vi "snap方式图像采集 1.vi"(8 "error in (no error)":errorcluster caption="错误输入（无错误）", 9 "Session In":T1, 10 "Image Name":string="I1") -> (0 "error out":errorcluster caption="错误输出", 2 "Session Out":T1, 3 "Image out":T2(plugin-control))   [LabVIEW 2017]
uses:
  <vilib>/userdefined/High Color/IMAQdx.ctl
  <vilib>/vision/driver/IMAQdx.llb/IMAQdx Camera Control Mode.ctl
  <vilib>/vision/driver/NI_Vision_Acquisition_Software.lvlib
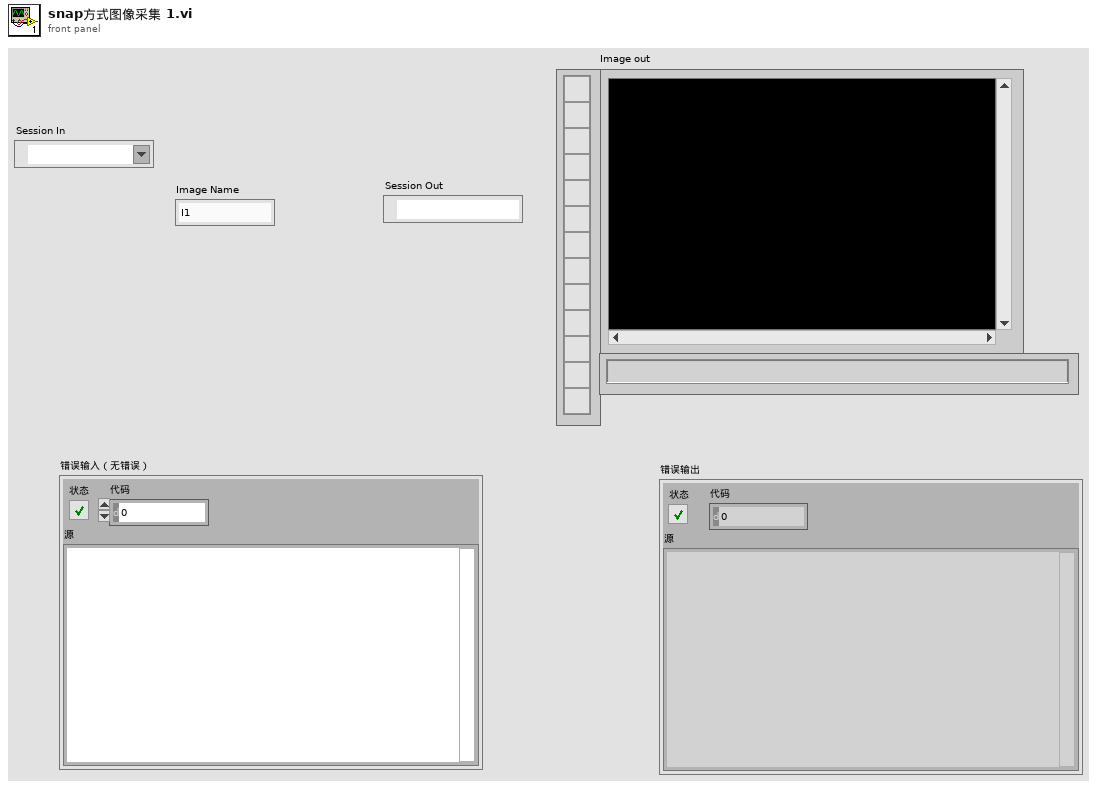
[diagram p1: front panel]
types:
  T1 = typedef "IMAQdx.ctl" = refnum<k21>
  T2 = typedef "IMAQ Image.ctl" = refnum<image>
  T3 = typedef "NI_Vision_Acquisition_Software.lvlib/IMAQdx Camera Control Mode.ctl" = enum32{"Controller", "Listener"}
  T4 = typedef "Image Type" = u32
  T5 = cluster{"IsNorImage":bool, "Exposure Values":u32, "ImagePath":path}
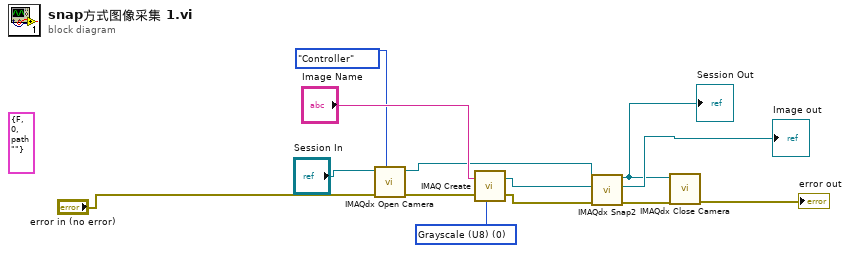
[diagram p0: block diagram]
diagram:
  w11 = T4 0 items=["Grayscale (U8)", "Grayscale (I16)", "Grayscale (SGL)", "Complex (CSG)", "RGB (U32)", "HSL (U32)", "RGB (U64)", "Grayscale (U16)"] ("Image Type")
  (unwired) T5 {"IsNorImage"=FALSE, "Exposure Values"=0, "ImagePath"=path ""} ("ParamsUI")
  n1 = call <vilib>:"IMAQdx Open Camera.vi"("Camera Control Mode"=IMAQdx_Camera_Control_Mode."Controller", "error in"="error in (no error)", "Session In"="Session In") -> ("error out"=w3:errorcluster, "Session Out"=w9:T1)  [unwired: 7 in]
  n2 = call "IMAQ Create"("Image Name"="Image Name", "Image Type"=w11, "error in (no error)"=w3) -> ("New Image"=w12:T2, "error out"=w2:errorcluster)  [unwired: 2 in]
  n3 = call <vilib>:"IMAQdx Snap2.vi"("error in"=w2, "Image In"=w12, "Session In"=w9) -> ("error out"=w7:errorcluster, "Image Out"=→"Image out":T2, "Session Out"=w5:T1)  [unwired: 6 in]
  "Session Out" <- w5
  n4 = call <vilib>:"IMAQdx Close Camera.vi"("error in"=w7, "Session In"=w5) -> ("error out"=→"error out":errorcluster)  [unwired: 9 in]
